vi "pumpsec_09.vi"(0 "reset":i32, 1 "master":i32, 2 "correction":dbl=1.0 format="%#_13g", 3 "manual":i32, 4 "pause":i32, 5 "Port":i32=10, 6 "pump_type":i32, 7 "port, Reglo D":i32, 10 "Target":dbl[](array[numeric])=[10.0, 2.0, 0.0, 0.0, 0.0, 0.0, 0.0, 0.0, 0.0, 0.0], 13 "Time":dbl[](array[numeric])=[4.0, 2.0, 0.0, 0.0, 0.0, 0.0, 0.0, 0.0, 0.0, 0.0], 16 "fr_manual":dbl) -> (11 "Reglo D":dbl, 14 "Scale":dbl, 15 "mA":dbl format="%#_2g", 17 "Scale actual":dbl, 18 "params":dbl[](array[numeric]), 19 "PAM":dbl)   [LabVIEW 2015]
uses:
  BERTTA.dll
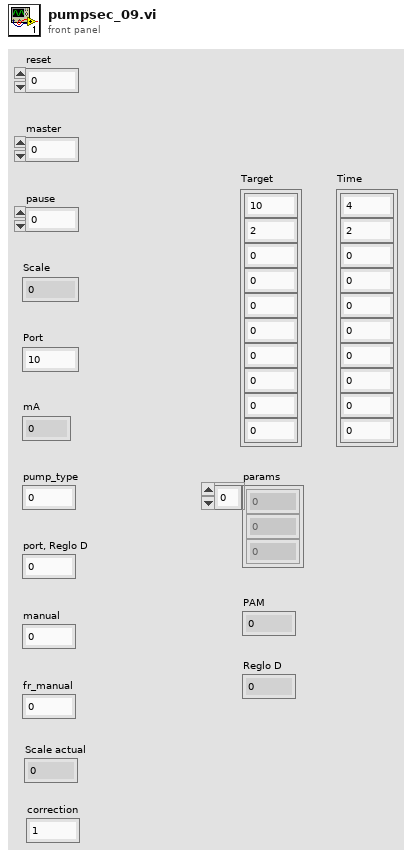
[diagram p1: front panel]
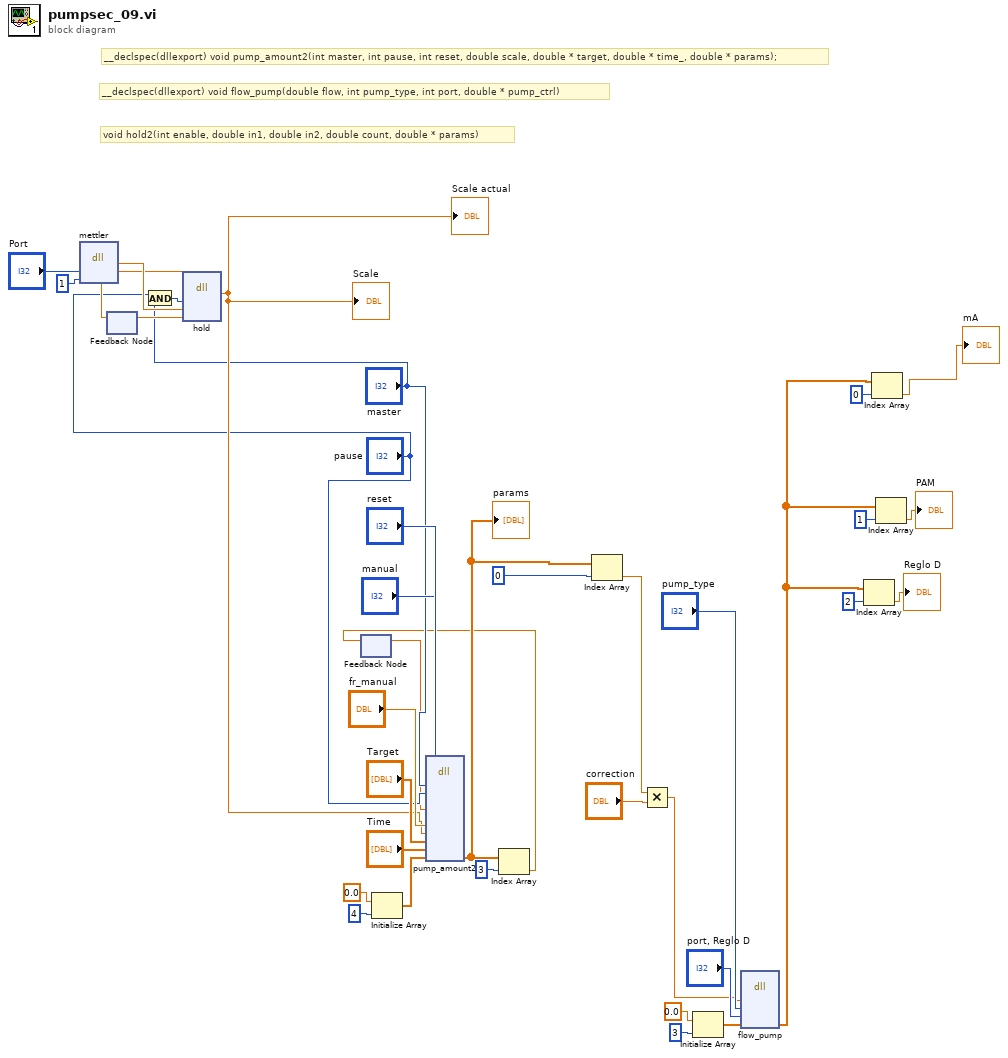
[diagram p0: block diagram]
diagram:
  # "void hold2(int enable, double in1, double in2, double count, double * params)"
  # "__declspec(dllexport) void flow_pump(double flow, int pump_type, int port, double * pump_ctrl)"
  # "__declspec(dllexport) void pump_amount2(int master, int pause, int reset, double scale, double * target, double * time_, double * params);"
  n1 = dll-call lib="C:/Users/shresplab/OneDrive - Kemira Oyj/Documents/Visual Studio 2017/Projects/Bertta/BERTTA/x64/Debug/BERTTA.dll" fn="mettler"("port"="Port", "msg"=1) -> ("return type"=w13:dbl)  [unwired: 5 in, 2 out]
  n2 = feedback #1() -> (w12:dbl)  [unwired: 1 in]
  n3 = And(x="pause", y="master") -> (x .and. y?=w8:i32)
  n4 = dll-call lib="C:/Users/shresplab/OneDrive - Kemira Oyj/Documents/Visual Studio 2017/Projects/Bertta/BERTTA/x64/Debug/BERTTA.dll" fn="hold"("enable"=w8, "in1"=w13, "in2"=w12) -> ("return type"=w11:dbl)  [unwired: 6 in, 2 out]
  "Scale" <- w11
  "Scale actual" <- w11
  n5 = feedback-in #1(w11) -> ()
  n6 = feedback #2() -> (w4:dbl)  [unwired: 1 in]
  n7 = Initialize Array(0.0 ("element"), 4 ("dimension size")) -> (w21:dbl[])
  n8 = dll-call lib="C:/Users/shresplab/OneDrive - Kemira Oyj/Documents/Visual Studio 2017/Projects/Bertta/BERTTA/x64/Debug/BERTTA.dll" fn="pump_amount2"("master"="master", "pause"="pause", "reset"="reset", "count"=w4, "manual"="manual", "fr_manual"="fr_manual", "scale"=w11, "target"="Target", "time_"="Time", "params"=w21) -> ("params"=w6:dbl[])  [unwired: 13 in, 2 out]
  "params" <- w6
  n9 = Index Array(array=w6, index=3) -> (element=w5:dbl)
  n10 = feedback-in #2(w5) -> ()
  n11 = Index Array(array=w6, index=0) -> (element=w3:dbl)
  n12 = Multiply(x=w3, y="correction") -> (x*y=w2:dbl)
  n13 = Initialize Array(0.0 ("element"), 3 ("dimension size")) -> (w26:dbl[])
  n14 = dll-call lib="C:/Users/shresplab/OneDrive - Kemira Oyj/Documents/Visual Studio 2017/Projects/Bertta/BERTTA/x64/Debug/BERTTA.dll" fn="flow_pump"("flow"=w2, "pump_type"="pump_type", "port"="port, Reglo D", "pump_ctrl"=w26) -> ("pump_ctrl"=w17:dbl[])  [unwired: 7 in, 2 out]
  n15 = Index Array(array=w17, index=2) -> (element=→"Reglo D":dbl)
  n16 = Index Array(array=w17, index=0) -> (element=→"mA":dbl)
  n17 = Index Array(array=w17, index=1) -> (element=→"PAM":dbl)
